vi "compress image to 65k_StateM.vi"(5 "Image":T1, 7 "error in (no error)":errorcluster) -> (0 "Data String":string, 3 "error out":errorcluster)   [LabVIEW 2011]
uses:
  IMAQ Image.ctl
  nivision.dll
panel:
  out "x*y":i32
  out "x/y":dbl(graph)
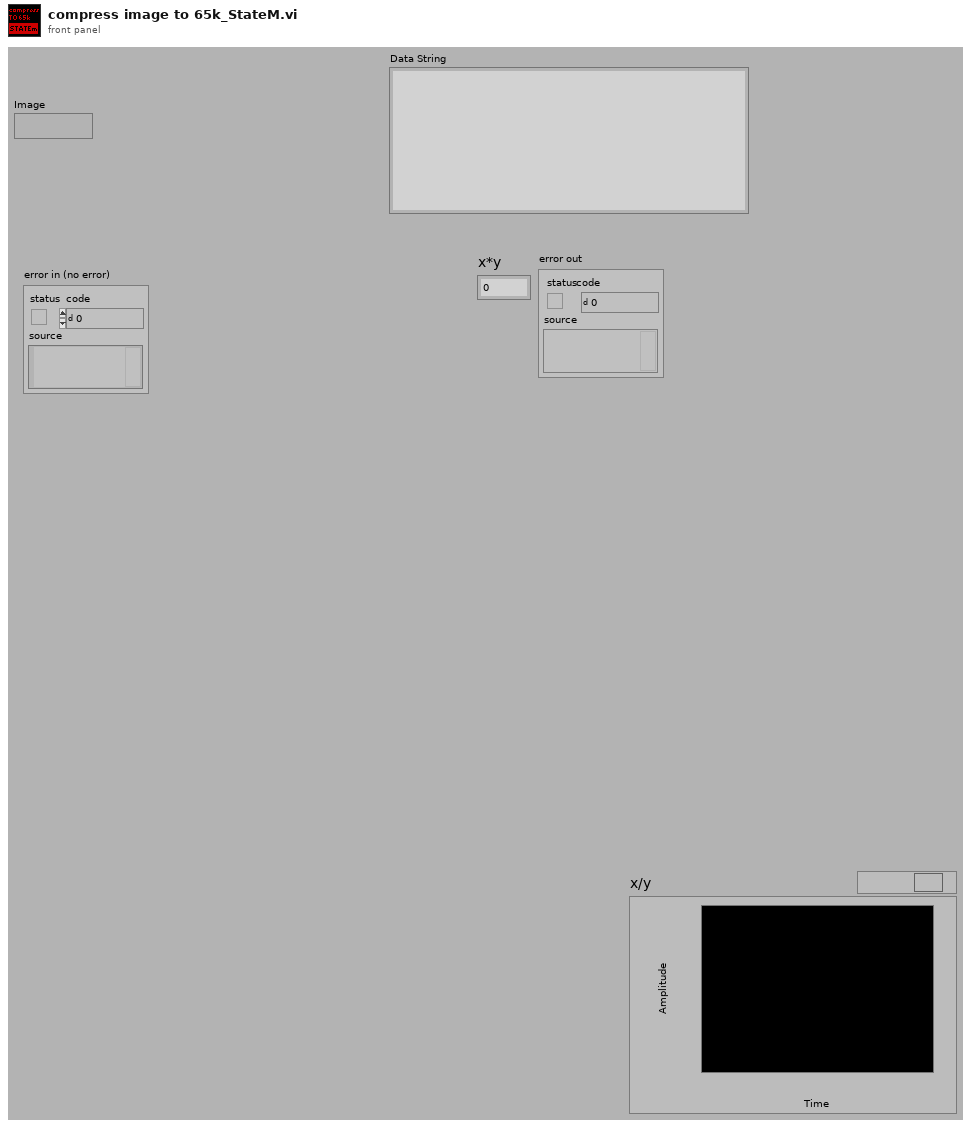
[diagram p1: front panel]
types:
  T1 = typedef "IMAQ Image.ctl" = refnum<image>
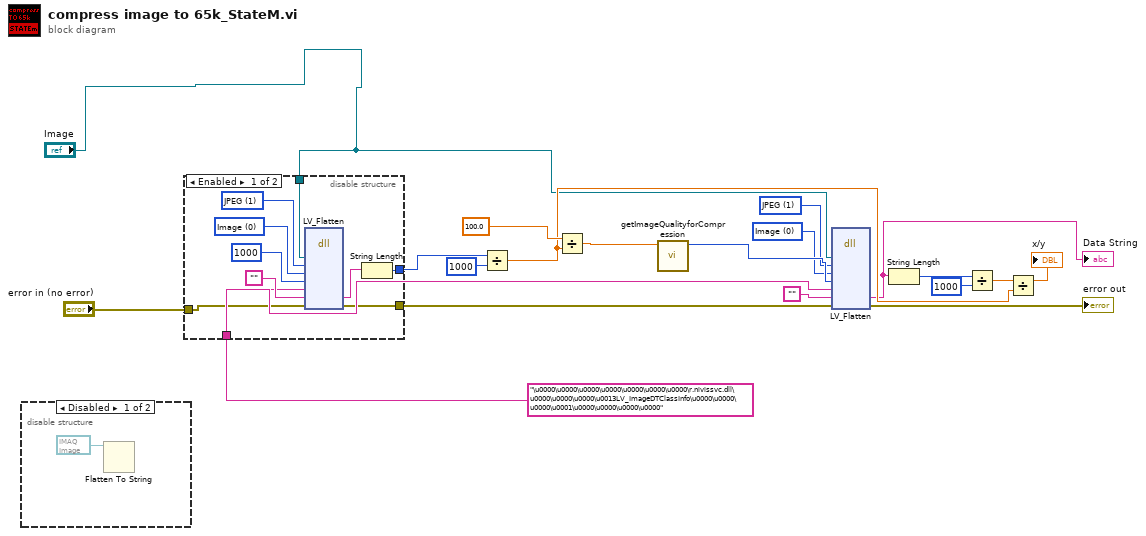
[diagram p0: block diagram]
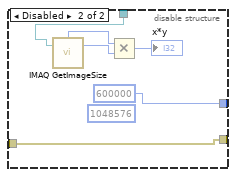
[diagram p2: hidden frame]
diagram:
  w5 = 0 items=["Image", "Image and Vision Info", "Reference to Image"] ("Type of Flatten (Image and Vision Info)")
  w4 = 1 items=["None", "JPEG", "PACKED BINARY"] ("Compression (None)")
  w8 = "\u0000\u0000\u0000\u0000\u0000\u0000\u0000\r.nivissvc.dll\u0000\u0000\u0000\u0013LV_ImageDTClassInfo\u0000\u0000\u0000\u0001\u0000\u0000\u0000\u0000" ("data string")
  n1 = disable-structure shown="Disabled" {
    frame Disabled {
      n2 = Flatten To String(anything=T1 refnum ("Image")) -> ()  [unwired: 1 in, 5 out]
    }
    frame Enabled {
    }
  }
  n3 = disable-structure shown="Enabled" {
    disable-tunnel: "Image" -> [w29 w34]
    disable-tunnel: "error in (no error)" -> [w28 w35]
    disable-tunnel: [w23 w35] -> w17
    disable-tunnel: w8 -> [w21 _]
    disable-tunnel: [w20 600000 ("Quality (750) 3")] -> w3
    frame Enabled {
      w26 = 0 items=["Image", "Image and Vision Info", "Reference to Image"] ("Type of Flatten (Image and Vision Info)")
      w27 = 1 items=["None", "JPEG", "PACKED BINARY"] ("Compression (None)")
      n4 = dll-call lib="nivision.*" fn="LV_Flatten"("Image"=w29, "compressionType"=w27, "flattenType"=w26, "quality"=1000 ("Quality (750) 3"), "data string"=w21, "output param"="", "error in (no error)"=w28) -> ("output param"=w22:string, "error in (no error)"=w23:errorcluster)  [unwired: 8 in, 3 out]
      n5 = String Length(string=w22) -> (length=w20:i32)
    }
    frame Disabled {
      (unwired) 1048576 ("x*y 2")
      n6 = call "IMAQ GetImageSize"("Image"=w34) -> ("Y Resolution"=w33:i32, "X Resolution"=w32:i32)  [unwired: 3 in, 1 out]
      n7 = Multiply(x=w32, y=w33) -> (x*y=→"x*y":i32)
    }
  }
  n8 = Divide(x=w3, y=1000) -> (x/y=w11:dbl)
  n9 = Divide(x=100.0 ("mean limit in kByte"), y=w11) -> (x/y=w10:dbl)
  n10 = call "getImageQualityforCompression.vi"("compression rate"=w10) -> ("quality"=w9:i16)  [unwired: 10 in]
  n11 = dll-call lib="nivision.*" fn="LV_Flatten"("Image"="Image", "compressionType"=w4, "flattenType"=w5, "quality"=w9, "data string"=w8, "output param"="", "error in (no error)"=w17) -> ("output param"=w7:string, "error in (no error)"=→"error out":errorcluster)  [unwired: 8 in, 3 out]
  "Data String" <- w7
  n12 = String Length(string=w7) -> (length=w16:i32)
  n13 = Divide(x=w16, y=1000) -> (x/y=w13:dbl)
  "x/y" <- w13
  n14 = Divide(x=w13, y=w11) -> ()  [unwired: 1 out]
